vi "Shutdown.vi"(8 "error in (no error)":errorcluster, 11 "Dispatcher in":refnum<class "Dispatcher.lvclass">) -> (0 "error out":errorcluster, 3 "Dispatcher out":refnum<class "Dispatcher.lvclass">)   [LabVIEW 2017, in "DSF Core.lvlib" / "Dispatcher.lvclass"]
uses:
  Dispatcher.lvclass
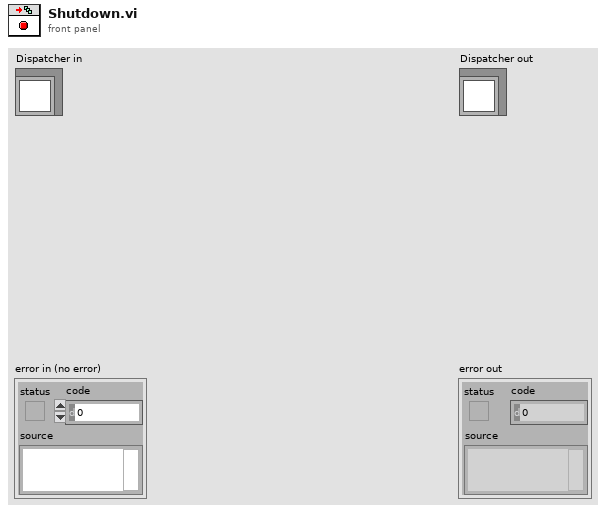
[diagram p1: front panel]
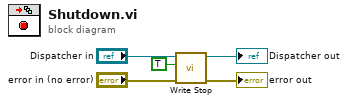
[diagram p0: block diagram]
diagram:
  n1 = call "Write Stop.vi"("error in (no error)"="error in (no error)", "stop"=TRUE, "Dispatcher in"="Dispatcher in") -> ("error out"=→"error out":errorcluster, "Dispatcher out"=→"Dispatcher out":refnum<class "Dispatcher.lvclass">)  [unwired: 7 in]
